vi "cascadeVelErrorPID.vi"(7 "PID gains":T1={"proportional gain (Kc)"=1.0, "integral time (Ti, min)"=0.01, "derivative time (Td, min)"=0.0} {"derivative time (Td, min)" format="%.3f"; "integral time (Ti, min)" format="%.3f"; "proportional gain (Kc)" format="%.3f"}, 8 "error in (no error)":errorcluster, 11 "Robot in":refnum<class "Robot.lvclass">) -> (0 "error out":errorcluster, 3 "Robot out":refnum<class "Robot.lvclass">)   [LabVIEW 2021, in "Robot.lvclass"]
uses:
  Robot.lvclass
  Robot.lvclass/Robot.ctl
  Read v_tang.vi
  Read v_norm.vi
  Read est_v_tang.vi
  Read est_v_norm.vi
  Write v_tang.vi
  Write v_norm.vi
  <vilib>/addons/control/pid/pid.llb/PID (DBL).vi
  <vilib>/addons/control/pid/NI_PID_pid.lvlib
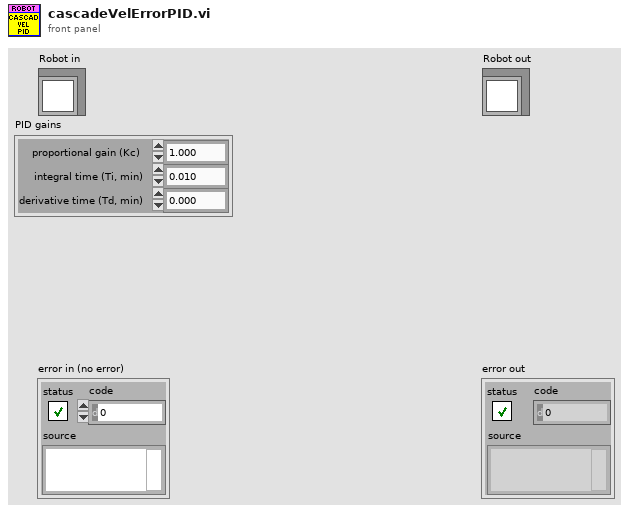
[diagram p1: front panel]
types:
  T1 = cluster{"proportional gain (Kc)":dbl, "integral time (Ti, min)":dbl, "derivative time (Td, min)":dbl}
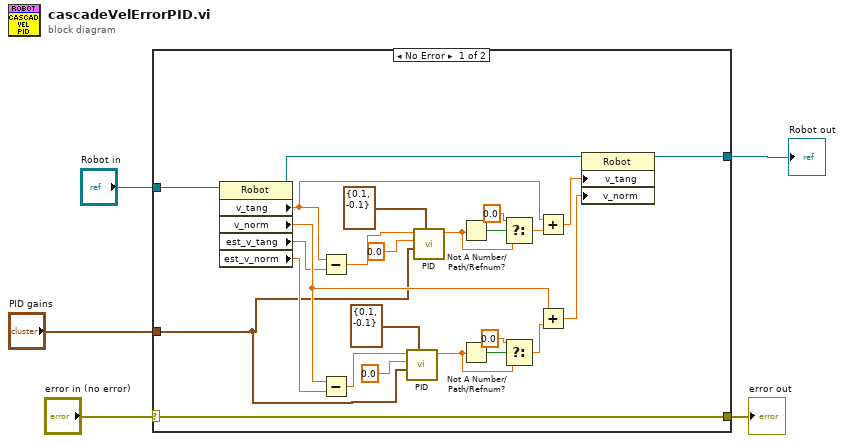
[diagram p0: block diagram]
diagram:
  n1 = case shown="No Error" "error in (no error)" {
    selector: "error in (no error)" -> [w30 w32]
    tunnel: [w30 w32] -> w4
    tunnel: [w15 w31] -> w2
    tunnel: "Robot in" -> [w16 w31]
    tunnel: "PID gains" -> [w8 _]
    frame No Error {
      n2 = property class="Robot"(reference=w16) -> (reference out=w29:refnum<class "Robot.lvclass">, "v_tang"=w25:dbl, "v_norm"=w26:dbl, "est_v_tang"=w24:dbl, "est_v_norm"=w28:dbl)  [unwired: 1 in, 1 out]
      n3 = Subtract(x=w25, y=w24) -> (x-y=w12:dbl)
      n4 = Subtract(x=w26, y=w28) -> (x-y=w10:dbl)
      n5 = call-poly <vilib>:"PID.vi"("output range"=cluster{"output high":dbl, "output low":dbl} {"output high"=0.1, "output low"=-0.1} ("Limits"), "PID gains"=w8, "process variable"=0.0 ("Setpoint"), "setpoint"=w10) -> ("output"=w6:dbl)  [unwired: 6 in, 1 out]
      n6 = call-poly <vilib>:"PID.vi"("output range"=cluster{"output high":dbl, "output low":dbl} {"output high"=0.1, "output low"=-0.1} ("Limits"), "PID gains"=w8, "process variable"=0.0 ("Setpoint"), "setpoint"=w12) -> ("output"=w7:dbl)  [unwired: 6 in, 1 out]
      n7 = Not A Number/Path/Refnum?(number/path/refnum=w7) -> (NaN/Path/Refnum?=w22:bool)
      n8 = Not A Number/Path/Refnum?(number/path/refnum=w6) -> (NaN/Path/Refnum?=w18:bool)
      n9 = Select(t=0.0, s=w22, f=w7) -> (s? t:f=w20:dbl)
      n10 = Select(t=0.0, s=w18, f=w6) -> (s? t:f=w17:dbl)
      n11 = Add(x=w25, y=w20) -> (x+y=w23:dbl)
      n12 = Add(x=w26, y=w17) -> (x+y=w27:dbl)
      n13 = property class="Robot"(reference=w29, "v_tang"=w23, "v_norm"=w27) -> (reference out=w15:refnum<class "Robot.lvclass">)  [unwired: 1 in, 1 out]
    }
    frame Error {
    }
  }
  "error out" <- w4
  "Robot out" <- w2
